vi "Read File Path.vi"(8 "error in (no error)":errorcluster, 11 "Log Open Message in":refnum<class "Log Open Message.lvclass">) -> (0 "error out":errorcluster, 2 "File Path":path, 3 "Log Open Message out":refnum<class "Log Open Message.lvclass">)   [LabVIEW 2017, in "Messaging.lvlib" / "Log Open Message.lvclass"]
uses:
  Log Open Message.lvclass
  Log Open Message.lvclass/Log Open Message.ctl
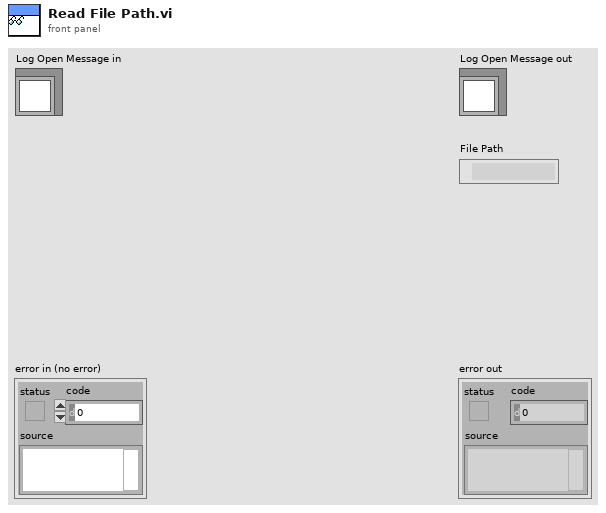
[diagram p1: front panel]
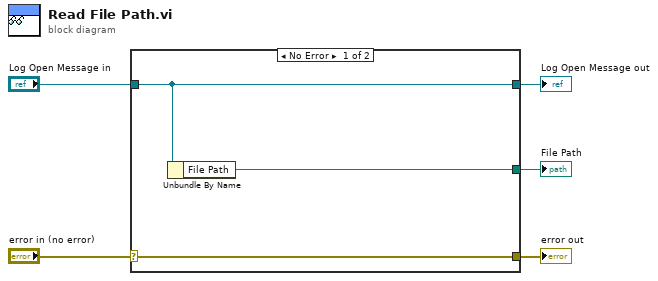
[diagram p0: block diagram]
diagram:
  n1 = case shown="No Error" "error in (no error)" {
    selector: "error in (no error)" -> [w8 w9]
    tunnel: [w8 w9] -> w4
    tunnel: [w7 w10] -> w2
    tunnel: "Log Open Message in" -> [w7 w10]
    tunnel: [w6 _] -> w1
    frame No Error {
      n2 = Unbundle By Name(w7) -> ("File Path"=w6:path)
    }
    frame Error {
    }
  }
  "error out" <- w4
  "Log Open Message out" <- w2
  "File Path" <- w1
